vi "TextDecorator_Create.vi"(8 "Error In":errorcluster, 10 "Text":refnum<class "IText.lvclass">, 11 "reference in":refnum<class "TextDecorator.lvclass">) -> (0 "Error Out":errorcluster, 3 "reference out":refnum<class "TextDecorator.lvclass">)   [LabVIEW 2024, in "TextDecorator.lvclass"]
uses:
  TextDecorator.lvclass
  TextDecorator.lvclass/TextDecorator.ctl
  IText/IText.lvclass
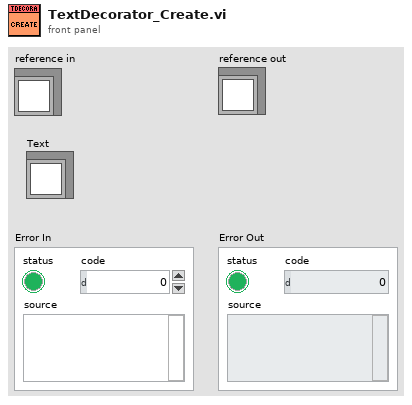
[diagram p1: front panel]
types:
  T1 = typedef "TextDecorator.lvclass/ObjectAttributes.ctl" = cluster{"TextRef":refnum<class "IText.lvclass">}
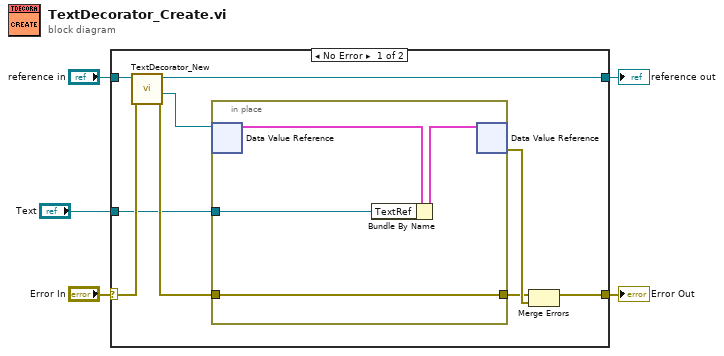
[diagram p0: block diagram]
diagram:
  n1 = case shown="No Error" "Error In" {
    selector: "Error In" -> [w13 w20]
    tunnel: [w7 w20] -> w4
    tunnel: "reference in" -> [w14 w19]
    tunnel: [w12 w19] -> w2
    tunnel: "Text" -> [w6 _]
    frame No Error {
      n2 = call "TextDecorator_New.vi"("Error In"=w13, "reference in"=w14) -> ("Error Out"=w9:errorcluster, "DVRRefOut"=w10:refnum<data-value>, "reference out"=w12:refnum<class "TextDecorator.lvclass">)  [unwired: 6 in, 1 out]
      n3 = in-place {
        in-place-border: w9 -> [w16]
        in-place-border: [w16] -> w8
        in-place-border: w6 -> [w15]
        n4 = in-place-dvr #1(w10) -> (w17:T1)  [unwired: 1 out]
        n5 = Bundle By Name(cluster=w17, "TextRef"=w15) -> (w18:T1)
        n6 = in-place-dvr #1(w18) -> (w11:errorcluster)  [unwired: 1 out]
      }
      n7 = Merge Errors(w8, w11) -> (w7:errorcluster)
    }
    frame Error {
      # "VI-TechBaseTemplate_Simple_4x4x4"
    }
  }
  "Error Out" <- w4
  "reference out" <- w2
